vi "bson_shared_empty.vi"() -> ()   [LabVIEW 2013]
uses:
  bson.ctl
panel:
  in  "bson":T1
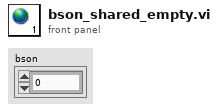
[diagram p1: front panel]
types:
  T1 = typedef "bson.ctl" = cluster{i32}
diagram:
